vi "Z -Stack Abort actions.vi"() -> (0 "error out":errorcluster)   [LabVIEW 2020]
uses:
  Typedefs/Read Write Enum.ctl
  Global Variables/FPGAstatus_Reference.vi
  <vilib>/Utility/error.llb/Error Cluster From Error Code.vi
  <vilib>/rvi/errors/niLvFpgaAdjustHostInterfaceError.vi
  <vilib>/rvi/interface/nirviReadWriteControl/nirviReadWriteControl.xnode
  RIG-SPECIFIC FILES/FPGA Refs/FPGA Ref.ctl
  NiFpgaLv.dll
  <vilib>/rvi/interface/Simulation/niFpgaSimulationCallBeginRW.vi
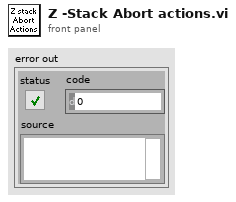
[diagram p1: front panel]
types:
  T1 = typedef "Read Write Enum.ctl" = enum16{"Read", "Write"}
  T2 = typedef "FPGA Ref.ctl" = refnum<k20>
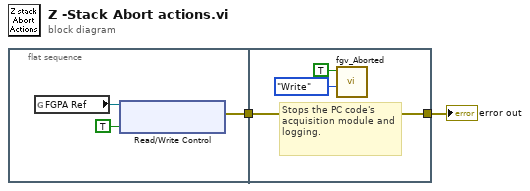
[diagram p0: block diagram]
diagram:
  n1 = flat-sequence {
    tunnel: [w3] -> w1
    tunnel: w1 -> [w6]
    tunnel: [w6] -> w2
    frame #0 {
      n2 = global read "FPGAstatus_Reference.vi" "FGPA Ref"() -> (w5:T2)
      n3 = xnode ("Read/Write Control")("FPGA VI Reference In"=w5, "ABORT Trig loop"=TRUE ("ABORT")) -> ("error out"=w3:errorcluster)  [unwired: 1 in, 1 out]
    }
    frame #1 {
      # "Stops the PC code's acquisition module and logging."
      n4 = call "fgv_Aborted.vi"("Function"=Read_Write_Enum."Write", "Funct Acq Aborted"=TRUE ("Aborted acquisition")) -> ()  [unwired: 8 in, 2 out]
    }
  }
  "error out" <- w2
